vi "initialize AO2 xy task.vi"(8 "error in (no error)":errorcluster, 11 "NI in":refnum<class "NI.lvclass">) -> (0 "error out":errorcluster, 3 "NI out":refnum<class "NI.lvclass">)   [LabVIEW 2021, in "NI.lvlib" / "NI.lvclass"]
uses:
  NI.lvclass
  NI.lvclass/NI.ctl
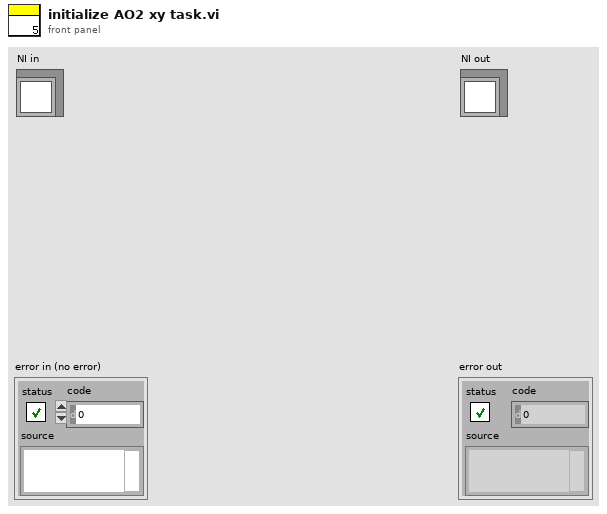
[diagram p1: front panel]
types:
  T1 = typedef "NI.lvlib/NI.lvclass/NI task parameters.ctl" = cluster{"exposure time":dbl, "camera H":dbl, "y line #":dbl, "flyback line #":dbl, "y pixel size":dbl, "z scan #":dbl, "z step size":dbl, "z offset":dbl, "laser all on?":bool, "laser option":bool[]}
  T2 = typedef "NI.lvlib/NI.lvclass/Channel Connection.ctl" = cluster{"Physical Channel":tag, "Terminal":tag, "StartTrigger":tag, "ClockSource":tag}
  T3 = cluster{"fast clock params":cluster{"fast clock rate":dbl, "off time after trigger":dbl, "cam line read time":dbl, "protect ticks #":dbl}, "AO1 laser Connection":T2, "AO2 zy Connection":T2, "AO3 z Connection (deprecated)":T2, "CO1 mainTrig Connection":T2, "CO2 fastClock Connection":T2, "AI phase Connection":T2}
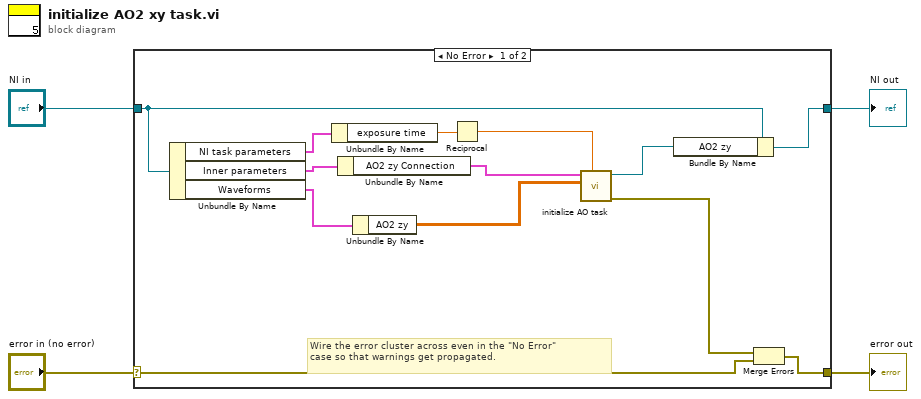
[diagram p0: block diagram]
diagram:
  n1 = case shown="No Error" "error in (no error)" {
    selector: "error in (no error)" -> [w7 w19]
    tunnel: [w6 w19] -> w3
    tunnel: [w12 w18] -> w1
    tunnel: "NI in" -> [w11 w18]
    frame No Error {
      # "Wire the error cluster across even in the \"No Error\"\ncase so that warnings get propagated."
      n2 = Unbundle By Name(w11) -> ("NI task parameters"=w10:T1, "Inner parameters"=w17:T3, "Waveforms"=w16:cluster{"AO1 laser":dbl[][], "AO2 zy":dbl[][]})
      n3 = Unbundle By Name(w10) -> ("exposure time"=w9:dbl)
      n4 = Unbundle By Name(w17) -> ("AO2 zy Connection"=w14:T2)
      n5 = Unbundle By Name(w16) -> ("AO2 zy"=w15:dbl[][])
      n6 = Reciprocal(x=w9) -> (1/x=w8:dbl)
      n7 = call "initialize AO task.vi"("rate"=w8, "waveform"=w15, "AO Connection"=w14) -> ("error out"=w5:errorcluster, "task out"=w13:refnum<k21>)  [unwired: 7 in]
      n8 = Bundle By Name(cluster=w11, "AO2 zy"=w13) -> (w12:refnum<class "NI.lvclass">)
      n9 = Merge Errors(w5, w7) -> (w6:errorcluster)
    }
    frame Error {
    }
  }
  "error out" <- w3
  "NI out" <- w1
